vi "Export Configuration RTM.vi"(8 "error in (no error)":errorcluster, 11 "Node Ptr":u64 format="%.0x") -> (0 "error out":errorcluster)   [LabVIEW 2020, in "Ballard MIL-STD-1553 System Explorer.lvlib" / "Implementation.lvlib"]
uses:
  Implementation.lvlib
  Scripting/Ballard MIL-STD-1553 Scripting.lvlib
panel:
  in  "Tag":string
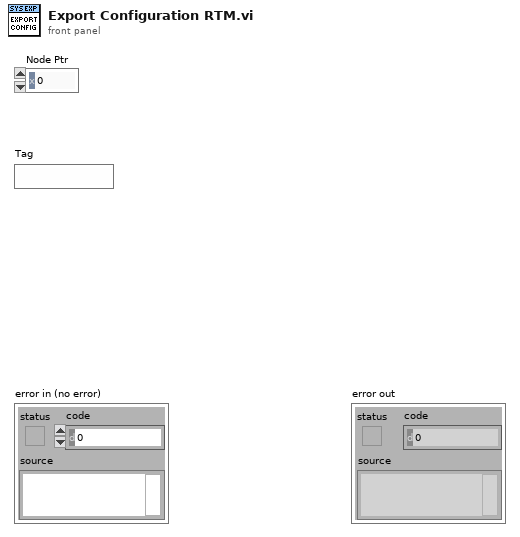
[diagram p1: front panel]
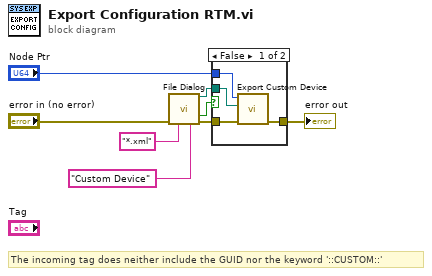
[diagram p0: block diagram]
diagram:
  # "The incoming tag does neither include the GUID nor the keyword '::CUSTOM::'"
  n1 = call "File Dialog"("error in"="error in (no error)", "pattern (all files)"="*.xml" ("pattern label"), "pattern label"="Custom Device") -> ("selected path"=w2:path, "cancelled"=w1:bool, "error out"=w4:errorcluster)  [unwired: 9 in, 1 out]
  n2 = case shown="False" w1 {
    tunnel: [w11 w13] -> w5
    tunnel: w4 -> [w12 w13]
    tunnel: "Node Ptr" -> [w10 _]
    tunnel: w2 -> [w9 _]
    frame False {
      n3 = call "Export Custom Device.vi"("error in"=w12, "path"=w9, "custom device ref in"=w10) -> ("error out"=w11:errorcluster)  [unwired: 7 in, 1 out]
    }
    frame True {
    }
  }
  "error out" <- w5
